vi "Find 3D Boundary.vi"(8 "Offset":i32, 9 "X":i32[](array[numeric]), 10 "Y":i32[](array[numeric]), 11 "Z":i32[](array[numeric])) -> (0 "Y Min":i32, 2 "X Min":i32, 3 "X Max":i32, 4 "Z Min":i32, 5 "Y Max":i32, 6 "Extreme Planes":cluster{"X":i32[], "Y":i32[], "Z":i32[]}, 7 "Z Max":i32)   [LabVIEW 2020, in "AoC 2022.lvlib"]
uses:
  AoC 2022.lvlib
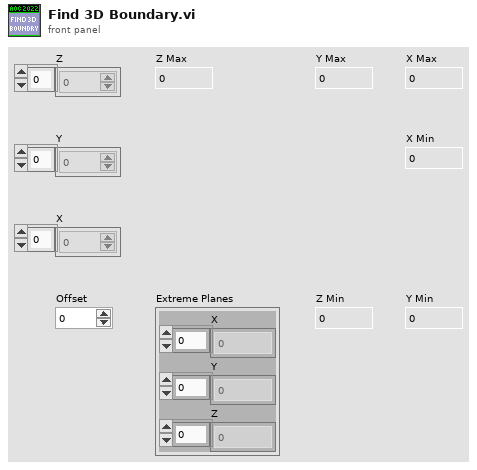
[diagram p1: front panel]
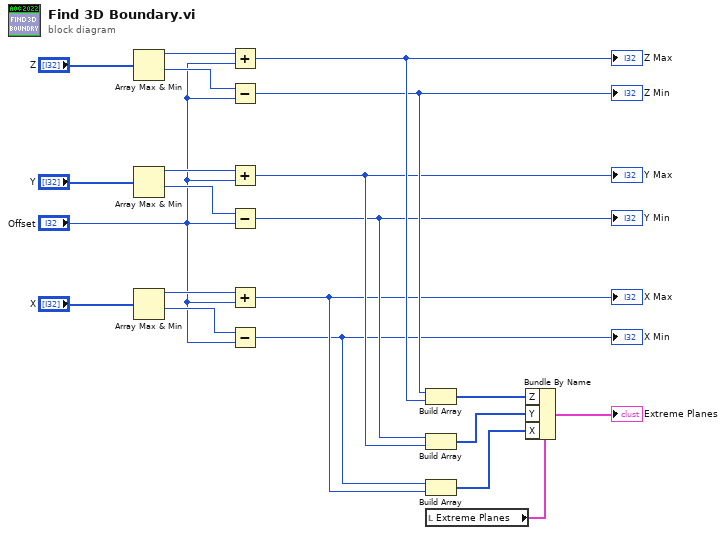
[diagram p0: block diagram]
diagram:
  n1 = Array Max & Min(array="Z") -> (max value=w13:i32, min value=w9:i32)  [unwired: 2 out]
  n2 = Array Max & Min(array="Y") -> (max value=w12:i32, min value=w8:i32)  [unwired: 2 out]
  n3 = Array Max & Min(array="X") -> (max value=w11:i32, min value=w10:i32)  [unwired: 2 out]
  n4 = Add(x=w13, y="Offset") -> (x+y=w6:i32)
  "Z Max" <- w6
  n5 = Subtract(x=w9, y="Offset") -> (x-y=w5:i32)
  "Z Min" <- w5
  n6 = Add(x=w12, y="Offset") -> (x+y=w4:i32)
  "Y Max" <- w4
  n7 = Subtract(x=w8, y="Offset") -> (x-y=w3:i32)
  "Y Min" <- w3
  n8 = Add(x=w11, y="Offset") -> (x+y=w2:i32)
  "X Max" <- w2
  n9 = Subtract(x=w10, y="Offset") -> (x-y=w1:i32)
  "X Min" <- w1
  n10 = Build Array(w5, w6) -> (w18:i32[])
  n11 = Build Array(w3, w4) -> (w17:i32[])
  n12 = Build Array(w1, w2) -> (w16:i32[])
  n13 = local read "Extreme Planes"() -> (w14:cluster{"X":i32[], "Y":i32[], "Z":i32[]})
  n14 = Bundle By Name(cluster=w14, "Z"=w18, "Y"=w17, "X"=w16) -> (→"Extreme Planes":cluster{"X":i32[], "Y":i32[], "Z":i32[]})
